vi "Change SystemLink Server for Local System.vi"(8 "error in (no error)":errorcluster, 11 "New SystemLink Server":string) -> (0 "error out":errorcluster)   [LabVIEW 2017]
uses:
  <vilib>/Utility/sysdir.llb/System Directory Type.ctl
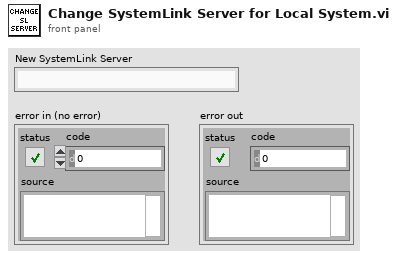
[diagram p1: front panel]
types:
  T1 = enum16{"open", "replace", "create", "open or create", "replace or create", "replace or create with confirmation"}
  T2 = typedef "System Directory Type.ctl" = i32
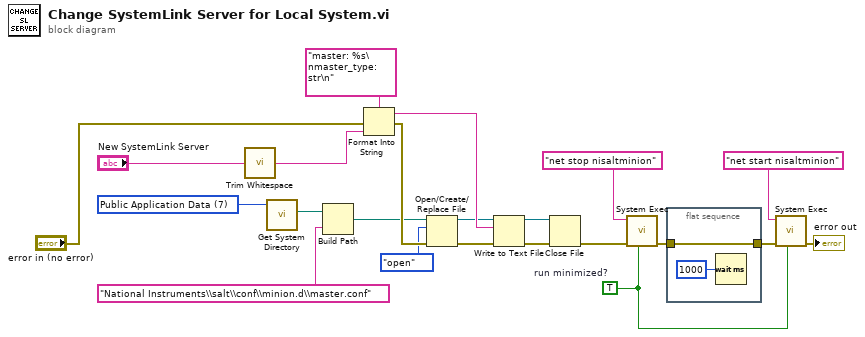
[diagram p0: block diagram]
diagram:
  w22 = TRUE  # run minimized?
  w1 = T2 7 items=["User Home"=0, "User Desktop"=1, "User Documents"=2, "User Application Data"=3, "User Preferences"=4, "User Temporary"=5, "Public Documents"=6, "Public Application Data"=7, "Public Preferences"=8, "Public Cache"=13, "System Core Libraries"=9, "System Installed Libraries"=10, "Application Files"=11, "Boot Volume Root"=12] ("system directory type")
  n1 = call <vilib>:"Trim Whitespace.vi"("string"="New SystemLink Server") -> ("trimmed string"=w9:string)  [unwired: 1 in]
  n2 = call <vilib>:"Get System Directory.vi"("system directory type"=w1) -> ("system directory"=w3:path)  [unwired: 10 in]
  n3 = Build Path(base path=w3, name or relative path="National Instruments\\salt\\conf\\minion.d\\master.conf") -> (appended path=w13:path)
  n4 = Format Into String(format string="master: %s\nmaster_type: str\n", error in="error in (no error)", w9) -> (resulting string=w6:string, error out=w14:errorcluster)  [unwired: 1 in]
  n5 = Open/Create/Replace File(file path (use dialog)=w13, error in=w14, operation (0:open)=T1."open") -> (refnum out=w5:refnum<file>, error out=w12:errorcluster)  [unwired: 3 in, 1 out]
  n6 = Write to Text File(file (use dialog)=w5, text=w6, error in=w12) -> (refnum out=w11:refnum<file>, error out=w10:errorcluster)  [unwired: 1 in, 1 out]
  n7 = Close File(refnum=w11, error in=w10) -> (error out=w16:errorcluster)  [unwired: 1 out]
  n8 = call <vilib>:"System Exec.vi"("run minimized? (F)"=w22, "error in (no error)"=w16, "command line"="net stop nisaltminion") -> ("error out"=w19:errorcluster)  [unwired: 5 in, 3 out]
  n9 = flat-sequence {
    tunnel: w19 -> [w24]
    tunnel: [w24] -> w20
    frame #0 {
      n10 = Wait (ms)(milliseconds to wait=u32 1000) -> ()  [unwired: 1 out]
    }
  }
  n11 = call <vilib>:"System Exec.vi"("run minimized? (F)"=w22, "error in (no error)"=w20, "command line"="net start nisaltminion") -> ("error out"=→"error out":errorcluster)  [unwired: 5 in, 3 out]
